vi "Pinouts.vi"(7 "JPG":refnum<vi>, 11 "Console Reference":refnum<vi>) -> ()   [LabVIEW 2021]
panel:
  in  "Tab Control":T1(tab)
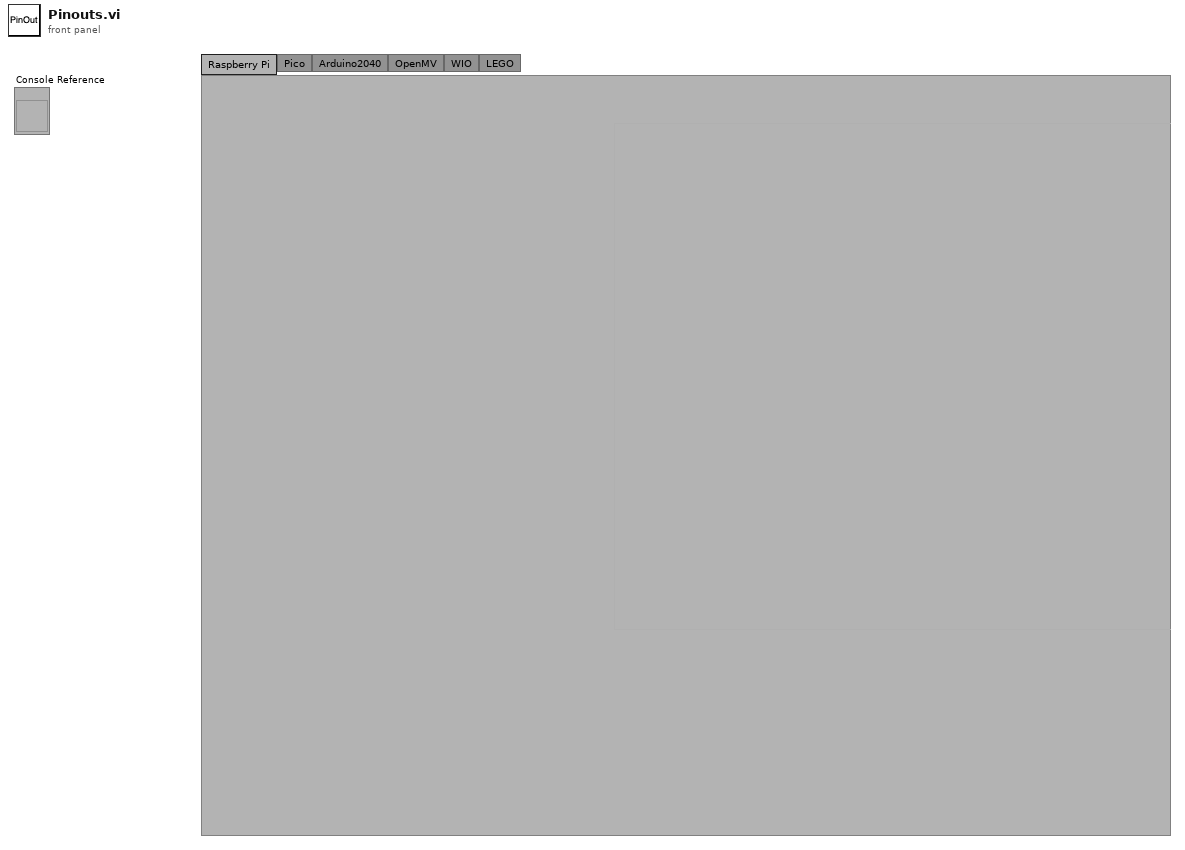
[diagram p1: front panel]
types:
  T1 = enum32{"Raspberry Pi", "Pico", "Arduino2040", "OpenMV", "WIO", "LEGO"}
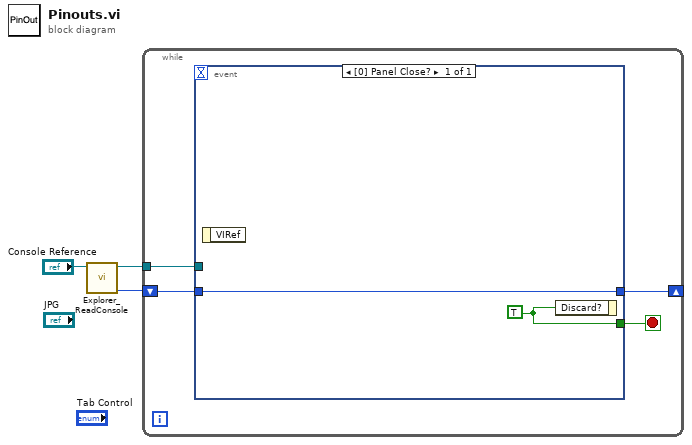
[diagram p0: block diagram]
diagram:
  n1 = call "Explorer_ReadConsole.vi"("String in"="Console Reference") -> ("index out"=w2:i32, "String out"=w1:refnum<vi>)  [unwired: 6 in, 3 out]
  n2 = while {
    shift-right: [w6] -> _
    shift-left: w2 -> [w5]
    tunnel: w1 -> [w4]
    stop <- w7 stop-if-true
    n3 = event shown="[0] Panel Close?" {
      selector: _ -> [_]
      dyn-events: _ -> [_]
      timeout: _ -> [_]
      tunnel: [w9] -> w7
      tunnel: [w8] -> w6
      tunnel: w5 -> [w8]
      tunnel: w4 -> [_]
      event Panel Close? {
        w9 = TRUE ("Discard?")
        n4 = event-data() -> ()  [unwired: 1 in, 1 out]
        n5 = event-data("Discard?"=w9) -> ()  [unwired: 1 in, 1 out]
      }
    }
  }
